vi "Main V2.vi"() -> ()   [LabVIEW 2019]
uses:
  States Enum.ctl
  Data Cluster.ctl
  <vilib>/express/express analysis/Spectral/Block/exnSpectralBlock spectral measurements RMS poly.vi
  <vilib>/express/express analysis/Spectral/Block/exnSpectralBlock spectral measurements RMS DDT.vi
  <vilib>/express/express analysis/Spectral/XNode/ExpressSpectralMeasurementsBlockNode.xnode
panel:
  out "Empty Channel":dynamicdata(graph)
  out "FFT 4":dynamicdata(graph)
  out "PZT Sensor":dynamicdata(graph)
  out "FFT 3":dynamicdata(graph)
  in  "Stop":bool
  in  "file path":path=path "C:/Users/lycan/OneDrive - The Ohio State University/Academics/Softwares/Labview/Frequency Analyzer/Frequency Analyzer Folder for LV19/OneDrive - The Ohio State University/Academics/Softwares/Labview/Frequency Analyzer/Test.xlsx.tdms"
  out "Drive Frequency (Hz)":dbl
  in  "Step Interval (ms)":dbl=100.0 min=0.2 max=5000000.0 step=0.1 format="%#.2p"
  in  "Step (Hz)":dbl=100.0 min=0.2 max=5000000.0 step=0.1 format="%#.2p"
  in  "Stop Frequency (Hz)":dbl=100.0 min=0.2 max=5000000.0 step=0.1 format="%#.2p"
  in  "Start Frequency(Hz)":dbl=100.0 min=0.2 max=5000000.0 step=0.1 format="%#.2p"
  in  "Amplitude (Vpp)":dbl=1.0 min=0.0 max=10.0 step=0.01 format="%#.2p"
  in  "Signal Route":u16(ring)=1 items=["Prototyping board", "FGEN BNC", "AO 0", "AO 1"]
  in  "Type":u16(ring) items=["Sine", "Triangle", "Square"]
  out "Microphone":dynamicdata(graph)
  out "FFT 2":dynamicdata(graph)
  out "FFT":dynamicdata(graph)
  out "PZT Actuator":dynamicdata(graph)
  # "Function Generator and Signal Analyzer"
  # "Error Message:"
  # "V 2.0"
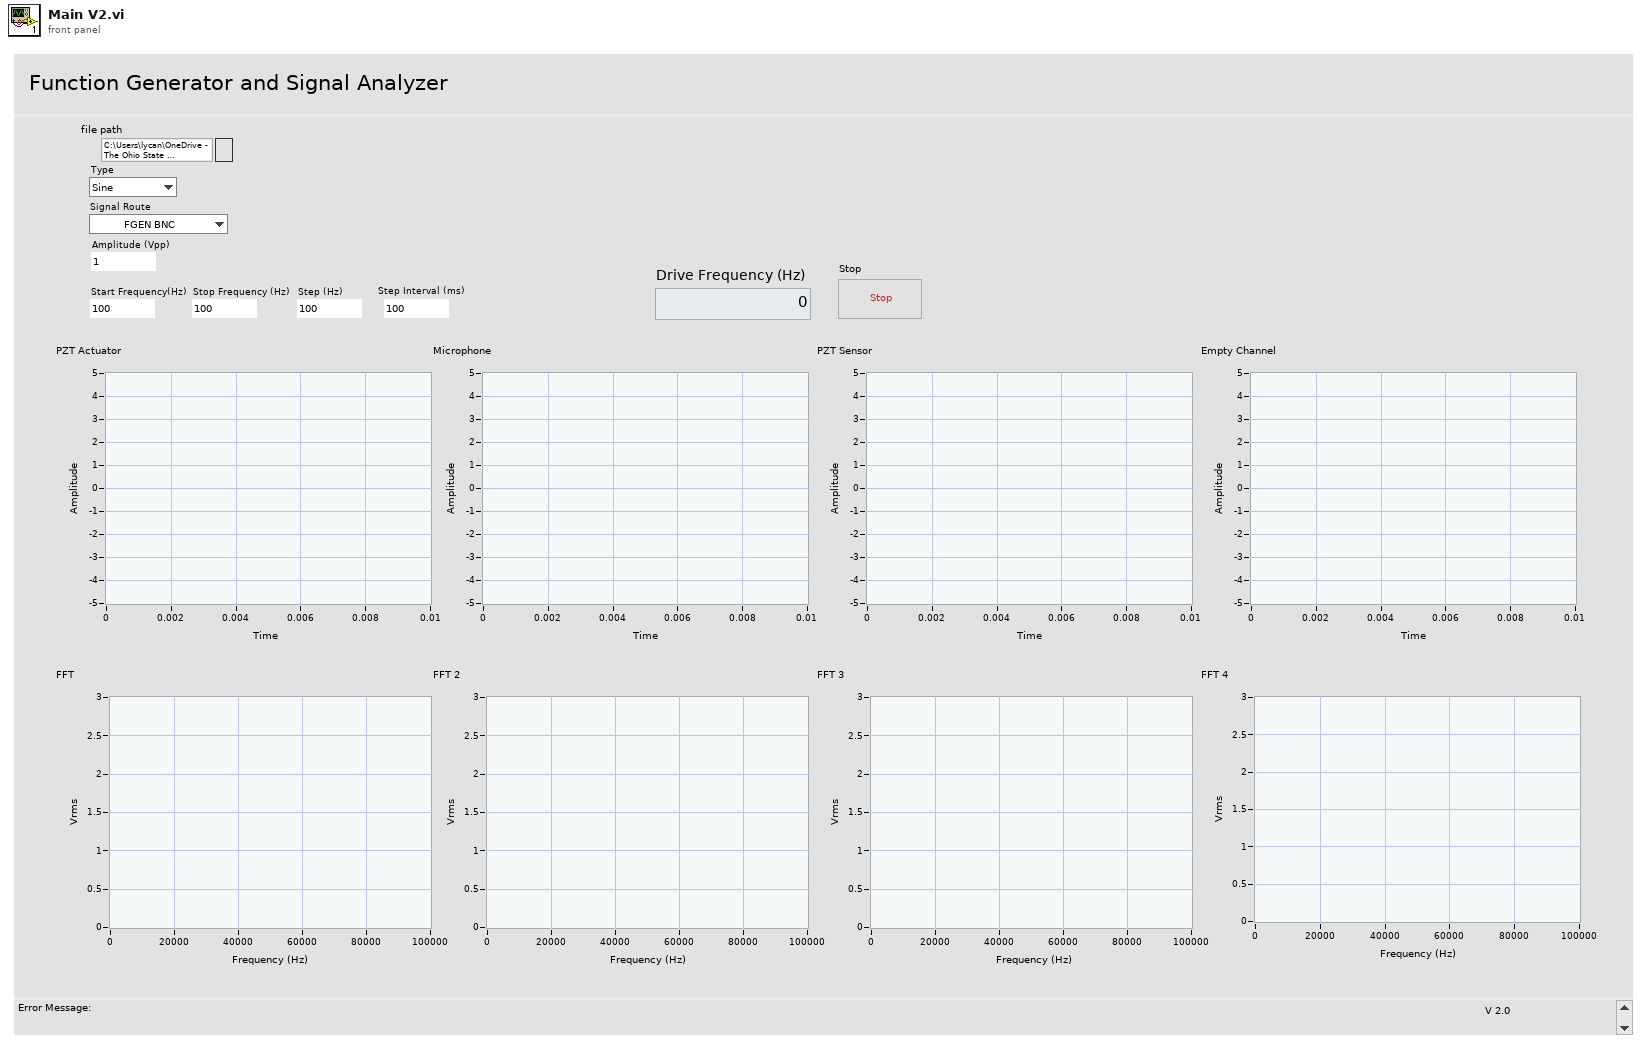
[diagram p1: front panel]
types:
  T1 = enum16{"open", "open or create", "create or replace", "create", "open (read-only)"}
  T2 = typedef "Data Cluster.ctl" = cluster{"Scope 1 Data":dbl[][], "Drive Frequency":dbl, "Scope 2 Data":dbl[][], "Scope 3 Data":dbl[][], "Scope 4 Data":dbl[][]}
  T3 = typedef "States Enum.ctl" = enum16{"Scope3", "Scope4", "Function Generator", "Scope1", "Scope2", "Stepping"}
  T4 = cluster{"averaging mode":u16, "weighting mode":u16, "number of averages":u32}
  T5 = cluster{"dB On (F)":bool, "unwrap phase (F)":bool, "convert to degree (F)":bool}
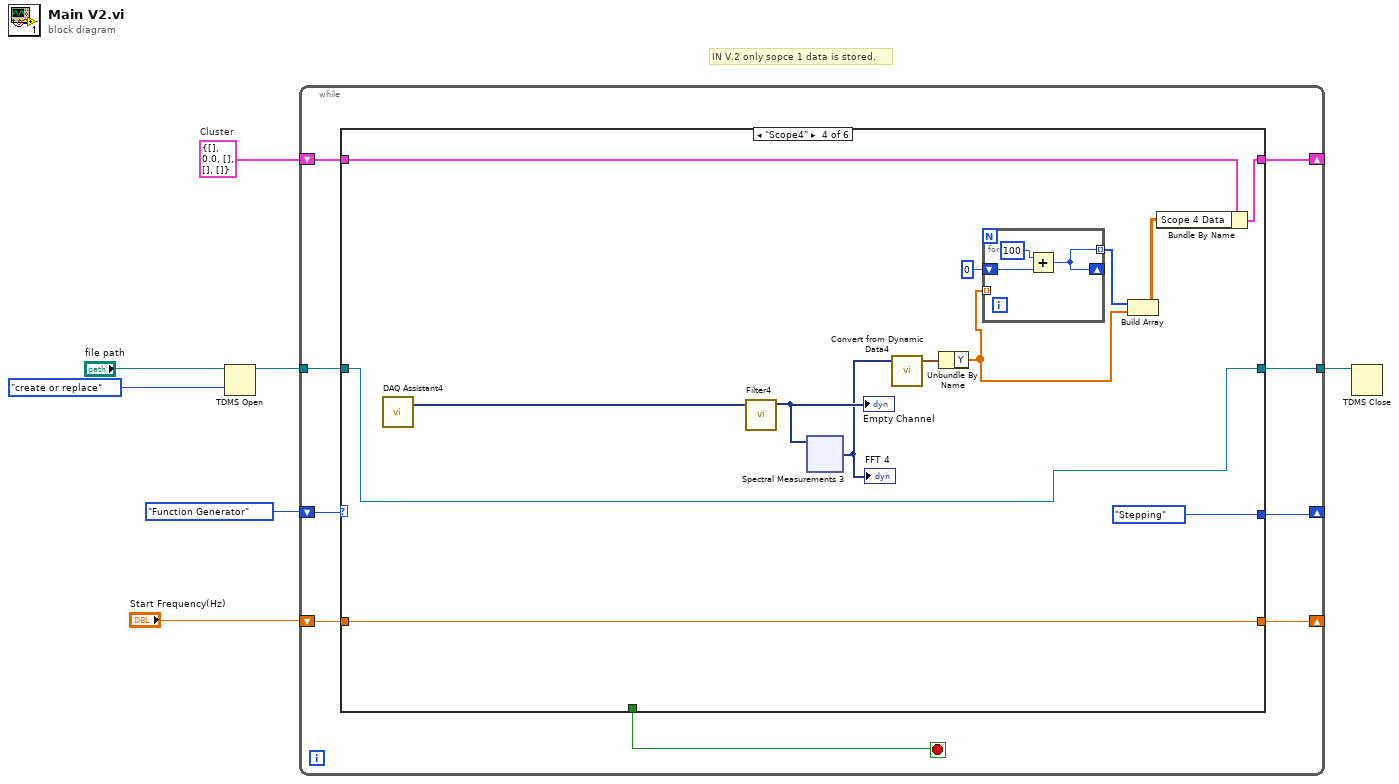
[diagram p0: block diagram]
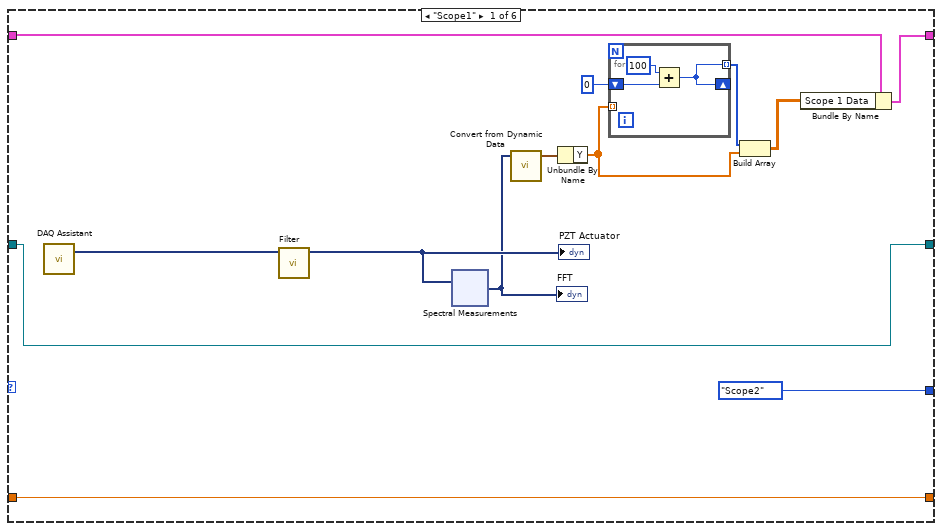
[diagram p2: hidden frame]
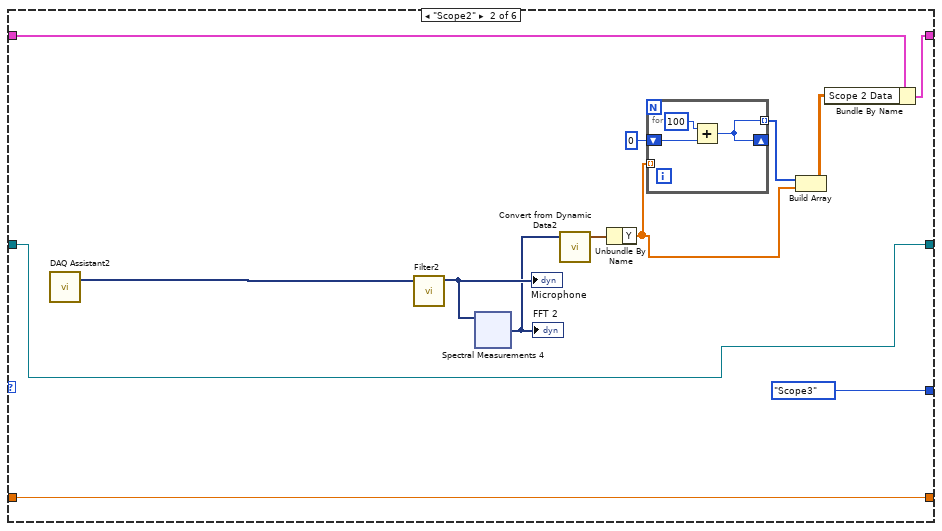
[diagram p3: hidden frame]
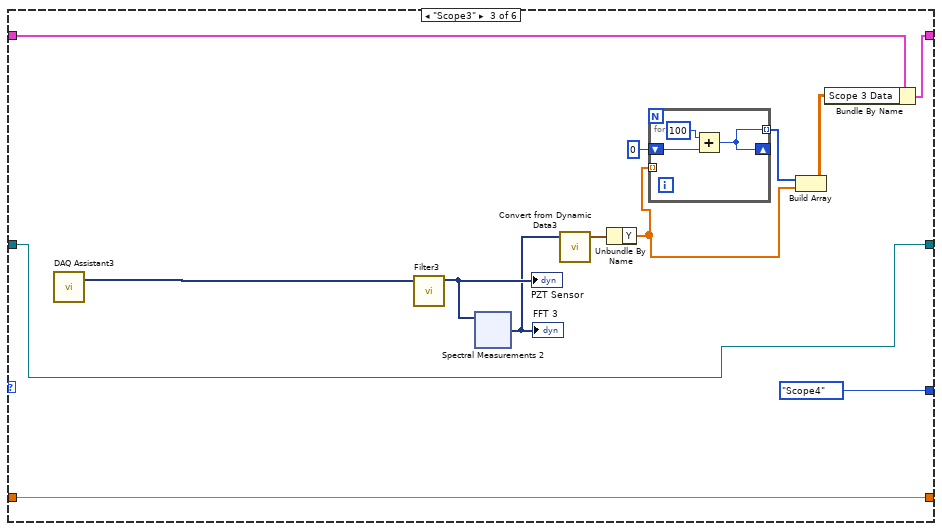
[diagram p4: hidden frame]
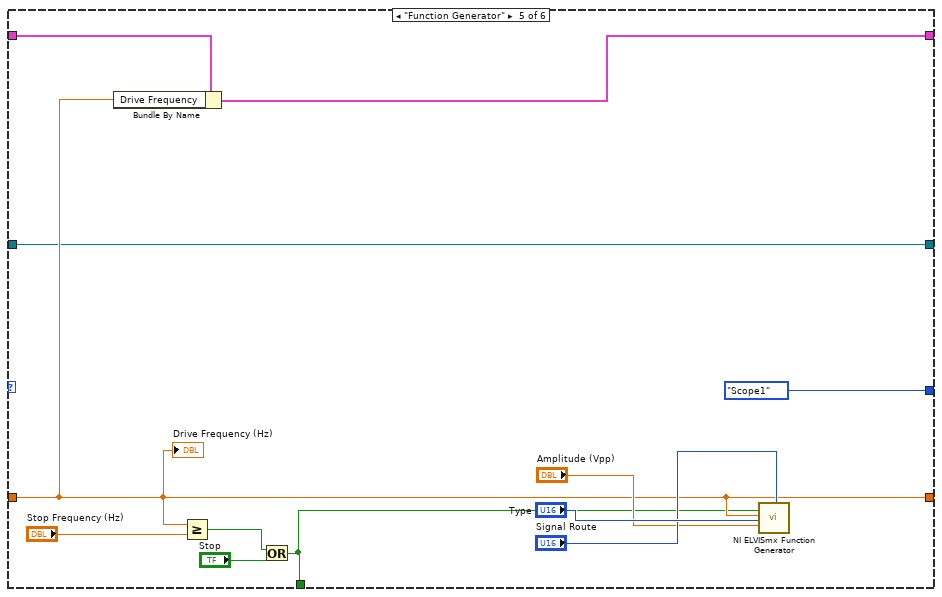
[diagram p5: hidden frame]
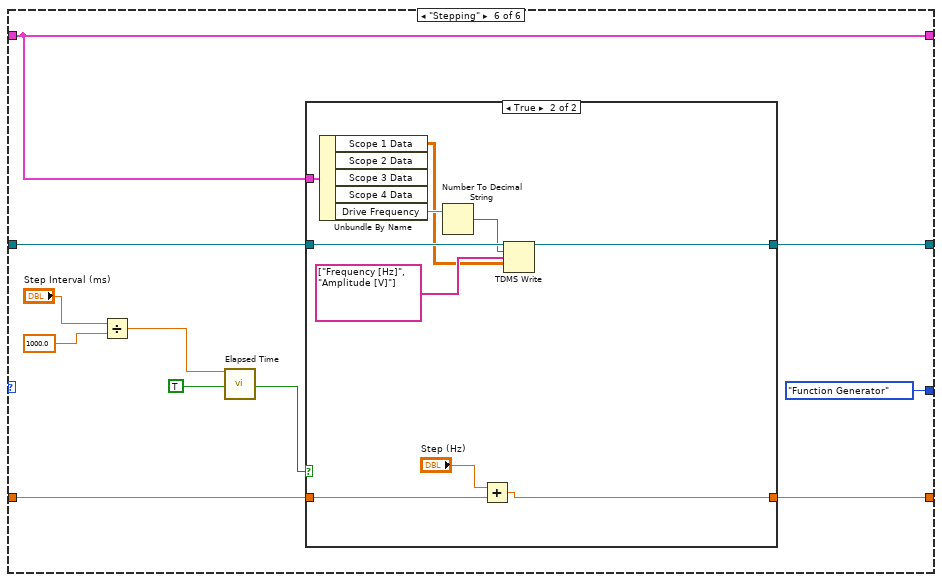
[diagram p6: hidden frame]
diagram:
  w5 = T2 {"Scope 1 Data"=[], "Drive Frequency"=0.0, "Scope 2 Data"=[], "Scope 3 Data"=[], "Scope 4 Data"=[]}  # Cluster
  # "IN V.2 only sopce 1 data is stored."
  n1 = TDMS Open(10:T1."create or replace" ("operation (0:open)"), 11:"file path") -> (3:w4:refnum<k34>)  [unwired: 5 in, 1 out]
  n2 = while {
    shift-right: [w16] -> _
    shift-left: States_Enum."Function Generator" ("Enum") -> [w15]
    shift-right: [w13] -> _
    shift-left: "Start Frequency(Hz)" -> [w14]
    shift-right: [w10] -> _
    shift-left: w5 -> [w11]
    tunnel: w4 -> [w9]
    tunnel: [w8] -> w3
    stop <- w12 stop-if-true
    n3 = case shown="\"Scope4\"" w15 {
      tunnel: [States_Enum."Scope2" ("Enum") States_Enum."Scope3" ("Enum") States_Enum."Scope4" ("Enum") States_Enum."Stepping" ("Enum") States_Enum."Scope1" ("Enum") States_Enum."Function Generator" ("Enum")] -> w16
      tunnel: w14 -> [w27 w53 w80 w107 w130 w145]
      tunnel: [w27 w53 w80 w107 w130 w140] -> w13
      tunnel: [_ _ _ _ w125 _] -> w12
      tunnel: w11 -> [w25 w50 w77 w104 w131 w137]
      tunnel: [w24 w47 w74 w101 w129 w137] -> w10
      tunnel: w9 -> [w22 w48 w75 w102 w128 w139]
      tunnel: [w22 w48 w75 w102 w128 w138] -> w8
      frame "Scope1" {
        n4 = call "DAQ Assistant"() -> ("data"=w29:dynamicdata)  [unwired: 17 in, 2 out]
        n5 = call "Filter"("Signal"=w29) -> ("Filtered Signal"=w21:dynamicdata)  [unwired: 9 in, 1 out]
        "PZT Actuator" <- w21
        n6 = xnode "Spectral Measurements"("Signals"=w21) -> ("FFT - (RMS)"=w20:dynamicdata)  [unwired: 2 in, 3 out]
        "FFT" <- w20
        n7 = call "Convert from Dynamic Data"("Dynamic Data Type"=w20) -> ("Waveform"=w26:waveform(dbl))  [unwired: 3 in]
        n8 = Unbundle By Name(w26) -> ("Y"=w19:dbl[])
        n9 = for {
          tunnel: w19 -> [_] mode=indexing
          tunnel: [w30] -> w17 mode=indexing
          shift-right: [w30] -> _
          shift-left: 0 -> [w31]
          n10 = Add(x=100, y=w31) -> (x+y=w30:i32)
        }
        n11 = Build Array(w17, w19) -> (w23:dbl[][])
        n12 = Bundle By Name(cluster=w25, "Scope 1 Data"=w23) -> (w24:T2)
      }
      frame "Scope2" {
        n13 = call "DAQ Assistant2"() -> ("data"=w55:dynamicdata)  [unwired: 17 in, 2 out]
        n14 = call "Filter2"("Signal"=w55) -> ("Filtered Signal"=w56:dynamicdata)  [unwired: 9 in, 1 out]
        "Microphone" <- w56
        n15 = xnode "Spectral Measurements 4"("Signals"=w56) -> ("FFT - (RMS)"=w51:dynamicdata)  [unwired: 2 in, 3 out]
        "FFT 2" <- w51
        n16 = call "Convert from Dynamic Data2"("Dynamic Data Type"=w51) -> ("Waveform"=w52:waveform(dbl))  [unwired: 3 in]
        n17 = Unbundle By Name(w52) -> ("Y"=w45:dbl[])
        n18 = for {
          tunnel: [w57] -> w44 mode=indexing
          shift-right: [w57] -> _
          shift-left: 0 -> [w58]
          tunnel: w45 -> [_] mode=indexing
          n19 = Add(x=100, y=w58) -> (x+y=w57:i32)
        }
        n20 = Build Array(w44, w45) -> (w49:dbl[][])
        n21 = Bundle By Name(cluster=w50, "Scope 2 Data"=w49) -> (w47:T2)
      }
      frame "Scope3" {
        n22 = call "DAQ Assistant3"() -> ("data"=w82:dynamicdata)  [unwired: 17 in, 2 out]
        n23 = call "Filter3"("Signal"=w82) -> ("Filtered Signal"=w83:dynamicdata)  [unwired: 9 in, 1 out]
        "PZT Sensor" <- w83
        n24 = xnode "Spectral Measurements 2"("Signals"=w83) -> ("FFT - (RMS)"=w78:dynamicdata)  [unwired: 2 in, 3 out]
        "FFT 3" <- w78
        n25 = call "Convert from Dynamic Data3"("Dynamic Data Type"=w78) -> ("Waveform"=w79:waveform(dbl))  [unwired: 3 in]
        n26 = Unbundle By Name(w79) -> ("Y"=w72:dbl[])
        n27 = for {
          tunnel: [w84] -> w73 mode=indexing
          shift-right: [w84] -> _
          shift-left: 0 -> [w85]
          tunnel: w72 -> [_] mode=indexing
          n28 = Add(x=100, y=w85) -> (x+y=w84:i32)
        }
        n29 = Build Array(w73, w72) -> (w76:dbl[][])
        n30 = Bundle By Name(cluster=w77, "Scope 3 Data"=w76) -> (w74:T2)
      }
      frame "Scope4" {
        n31 = call "DAQ Assistant4"() -> ("data"=w109:dynamicdata)  [unwired: 17 in, 2 out]
        n32 = call "Filter4"("Signal"=w109) -> ("Filtered Signal"=w110:dynamicdata)  [unwired: 9 in, 1 out]
        "Empty Channel" <- w110
        n33 = xnode "Spectral Measurements 3"("Signals"=w110) -> ("FFT - (RMS)"=w105:dynamicdata)  [unwired: 2 in, 3 out]
        "FFT 4" <- w105
        n34 = call "Convert from Dynamic Data4"("Dynamic Data Type"=w105) -> ("Waveform"=w106:waveform(dbl))  [unwired: 3 in]
        n35 = Unbundle By Name(w106) -> ("Y"=w98:dbl[])
        n36 = for {
          tunnel: [w111] -> w99 mode=indexing
          shift-right: [w111] -> _
          shift-left: 0 -> [w112]
          tunnel: w98 -> [_] mode=indexing
          n37 = Add(x=100, y=w112) -> (x+y=w111:i32)
        }
        n38 = Build Array(w99, w98) -> (w103:dbl[][])
        n39 = Bundle By Name(cluster=w104, "Scope 4 Data"=w103) -> (w101:T2)
      }
      frame "Function Generator" {
        n40 = Bundle By Name(cluster=w131, "Drive Frequency"=w130) -> (w129:T2)
        n41 = Greater Or Equal?(x=w130, y="Stop Frequency (Hz)") -> (x >= y?=w127:bool)
        n42 = Or(x=w127, y="Stop") -> (x .or. y?=w125:bool)
        n43 = call "NI ELVISmx Function Generator"("Stop"=w125, "Frequency (Hz)"=w130, "Amplitude (Vpp)"="Amplitude (Vpp)", "Type"="Type", "Signal Route"="Signal Route") -> ()  [unwired: 13 in, 2 out]
        "Drive Frequency (Hz)" <- w130
      }
      frame "Stepping" {
        n44 = Divide(x="Step Interval (ms)", y=1000.0) -> (x/y=w142:dbl)
        n45 = call "Elapsed Time"("Time Target (s)"=w142, "Auto Reset"=TRUE) -> ("Time has Elapsed"=w146:bool)  [unwired: 10 in, 7 out]
        n46 = case shown="True" w146 {
          tunnel: w145 -> [w149 w158]
          tunnel: [w149 w157] -> w140
          tunnel: w137 -> [_ w156]
          tunnel: w139 -> [w148 w153]
          tunnel: [w148 w150] -> w138
          frame False {
          }
          frame True {
            n47 = Unbundle By Name(w156) -> ("Scope 1 Data"=w152:dbl[][], "Drive Frequency"=w155:dbl)  [unwired: 3 out]
            n48 = Number To Decimal String(number=w155) -> (decimal integer string=w151:string)  [unwired: 1 in]
            n49 = Add(x="Step (Hz)", y=w158) -> (x+y=w157:dbl)
            n50 = TDMS Write(0:w153, 5:w151, 7:string[] ["Frequency [Hz]", "Amplitude [V]"] ("channel name(s) in (Untitled)"), 9:w152) -> (4:w150:refnum<k34>)  [unwired: 2 in, 3 out]
          }
        }
      }
    }
  }
  n51 = TDMS Close(11:w3) -> ()  [unwired: 1 in, 2 out]
